vi "LVITX 2D X&Y Commands.vi"(1 "Kill X&Y waves?":bool=TRUE, 2 "Y wave":string, 3 "X wave":string, 4 "2D wave":string) -> (0 "result string":string)   [LabVIEW 2011]
panel:
  in  "input string 2":string="KillWaves #waveX#\nKillWaves #waveY#"
  in  "input string 1":string="SetScale/I x #waveX#[0],#waveX#[DimSize(#waveX#, 0)],\"\", '#wave2D#'\nSetScale/I y #waveY#[0],#waveY#[DimSize(#waveY#, 0)],\"\", '#wave2D#'\n"
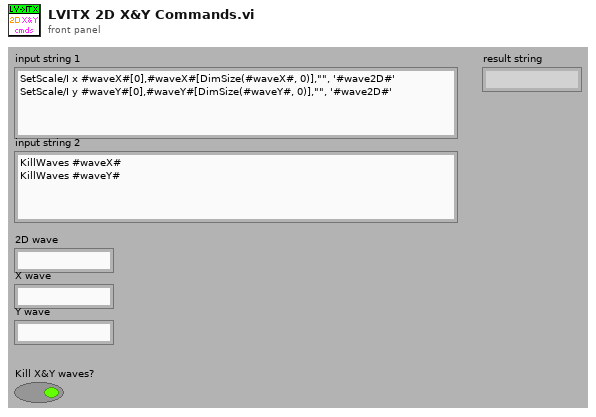
[diagram p1: front panel]
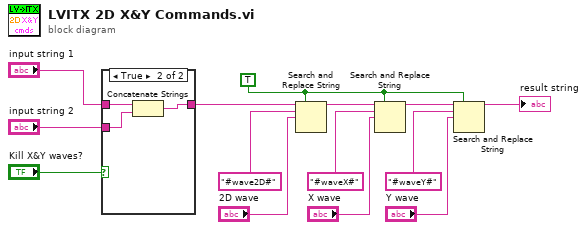
[diagram p0: block diagram]
diagram:
  w10 = TRUE ("replace all? (F)")
  n1 = case shown="True" "Kill X&Y waves?" {
    tunnel: "input string 1" -> [w15 w18]
    tunnel: [w15 w17] -> w3
    tunnel: "input string 2" -> [_ w16]
    frame False {
    }
    frame True {
      n2 = Concatenate Strings(w18, w16) -> (w17:string)
    }
  }
  n3 = Search and Replace String(replace all?=w10, input string=w3, search string="#wave2D#", replace string="2D wave") -> (result string=w5:string)  [unwired: 1 in, 6 out]
  n4 = Search and Replace String(replace all?=w10, input string=w5, search string="#waveX#", replace string="X wave") -> (result string=w7:string)  [unwired: 1 in, 6 out]
  n5 = Search and Replace String(replace all?=w10, input string=w7, search string="#waveY#", replace string="Y wave") -> (result string=→"result string":string)  [unwired: 1 in, 6 out]
